vi "Rubbish.vi"() -> ()   [LabVIEW 2014]
uses:
  <vilib>/myRIO/Common/Instrument Driver Framework/myRIO v1.0/DIO/typedefs/DIO Channels Enum.ctl
  <vilib>/myRIO/Common/Instrument Driver Framework/myRIO v1.0/DIO/typedefs/DIO Channels List.ctl
  <vilib>/myRIO/Common/Instrument Driver Framework/Utilities/typedefs/Generic FPGA Reference.ctl
  <vilib>/myRIO/Common/Instrument Driver Framework/Utilities/typedefs/myRIO v1.0 Reference.ctl
  <vilib>/myRIO/Common/Instrument Driver Framework/Utilities/typedefs/Hardware Version Enum.ctl
  <vilib>/myRIO/Common/Instrument Driver Framework/Utilities/typedefs/myRIO Generic Hardware Reference.ctl
  <vilib>/myRIO/Instrument Drivers/Onboard IO/DIO/typedefs/DIO Reference.ctl
  <vilib>/myRIO/Instrument Drivers/Onboard IO/DIO/DIO.lvlib
  <vilib>/myRIO/Instrument Drivers/Onboard IO/DIO/vis/Read.vi
  <vilib>/userdefined/High Color/nirio_resource_hc.ctl
  <vilib>/myRIO/Common/Instrument Driver Framework/myRIO v1.0/DIO/vis/myRIO v1.1 Open DIO.vi
  <vilib>/myRIO/Instrument Drivers/Onboard IO/DIO/vis/myRIO DIO Open.xnode
  <vilib>/myRIO/Common/Instrument Driver Framework/Utilities/vis/Is FPGA Ref Available.vi
  <vilib>/myRIO/Express VI/Onboard IO/DI/DI Express VI.xnode
  <vilib>/functionblocks/Edge Detection/One Shot Falling With Input/One Shot Falling With Input.vi
  <vilib>/functionblocks/NI_FunctionBlock Libraries.lvlib
  <vilib>/functionblocks/FB Core/FB Core.xnode
  <vilib>/myRIO/Instrument Drivers/Onboard IO/DIO/vis/Write.vi
  <vilib>/myRIO/Express VI/Onboard IO/DO/DO Express VI.xnode
  <vilib>/myRIO/Instrument Drivers/Utilities/Utilities.lvlib
panel:
  in  "stop":bool
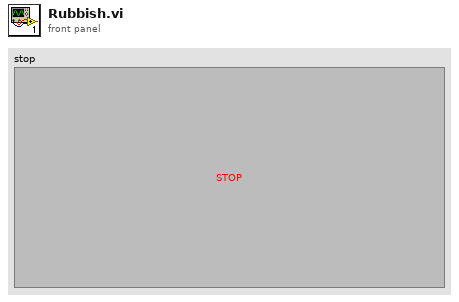
[diagram p1: front panel]
types:
  T1 = typedef "DIO.lvlib/DIO Reference.ctl" = cluster{"myRIO Reference":T2, "DIO Channels List":T6}
  T2 = typedef "myRIO Generic Hardware Reference.ctl" = cluster{"myRIO Model":T3, "myRIO Hardware Reference":T4}
  T3 = typedef "Hardware Version Enum.ctl" = enum16{"Unknown", "myRIO-1900", "myRIO-1950"}
  T4 = typedef "myRIO v1.0 Reference.ctl" = cluster{"Generic FPGA Reference":T5, "Allow multiple opens":bool}
  T5 = typedef "Generic FPGA Reference.ctl" = refnum<k20>
  T6 = typedef "DIO Channels List.ctl" = T7[]
  T7 = typedef "DIO Channels Enum.ctl" = enum16{"Not Connected", "C/DIO0", "C/DIO1", "C/DIO2", "C/DIO3", "C/DIO4", "C/DIO5", "C/DIO6", "C/DIO7", "A/DIO0", "A/DIO1", "A/DIO2", "A/DIO3", "A/DIO4", "A/DIO5", "A/DIO6", "A/DIO7", "A/DIO8", "A/DIO9", "A/DIO10", "A/DIO11", "A/DIO12", "A/DIO13", "A/DIO14", "A/DIO15", "B/DIO0", "B/DIO1", "B/DIO2", "B/DIO3", "B/DIO4", "B/DIO5", "B/DIO6", "B/DIO7", "B/DIO8", "B/DIO9", "B/DIO10", "B/DIO11", "B/DIO12", "B/DIO13", "B/DIO14", "B/DIO15", "LED0", "LED1", "LED2", "LED3", "Button0"}
  T8 = typedef "nirio_resource_hc.ctl" = tag
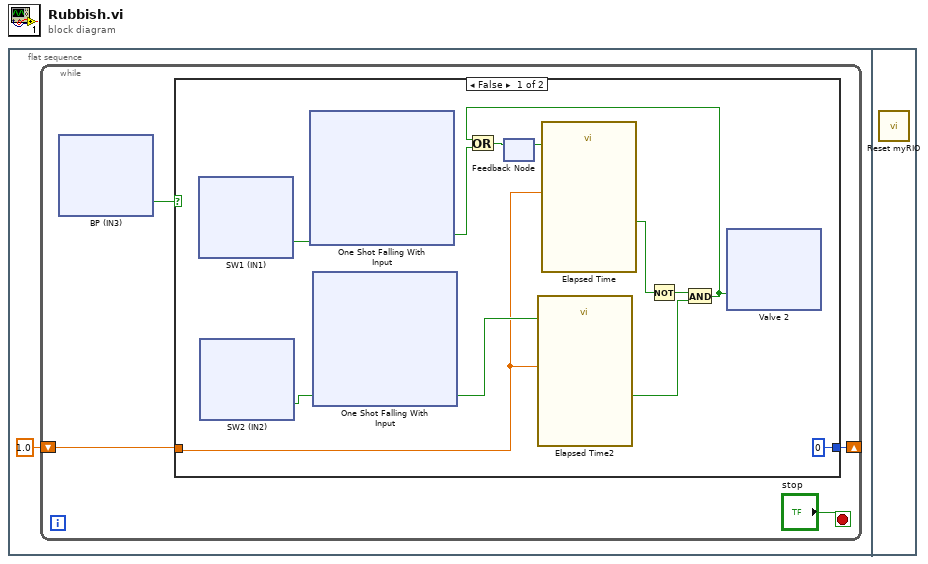
[diagram p0: block diagram]
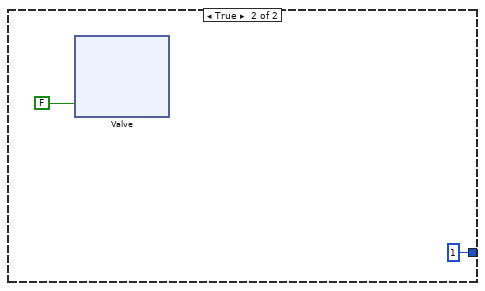
[diagram p2: hidden frame]
diagram:
  n1 = flat-sequence {
    frame #0 {
      n2 = while {
        shift-right: [w2] -> _
        shift-left: 1.0 -> [w3]
        stop <- "stop" stop-if-true
        n3 = xnode "BP (IN3)"() -> ("B/DIO1 (Pin 13)"=w4:bool)  [unwired: 1 in, 1 out]
        n4 = case shown="False" w4 {
          tunnel: w3 -> [w8 _]
          tunnel: [0 1] -> w2
          frame False {
            n5 = xnode "SW1 (IN1)"() -> ("B/DIO5 (Pin 21)"=w9:bool)  [unwired: 1 in, 1 out]
            n6 = xnode "SW2 (IN2)"() -> ("B/DIO2 (Pin 15)"=w17:bool)  [unwired: 1 in, 1 out]
            n7 = xnode "One Shot Falling With Input"("input"=w9) -> ("output"=w10:bool)  [unwired: 1 in, 1 out]
            n8 = xnode "One Shot Falling With Input"("input"=w17) -> ("output"=w14:bool)  [unwired: 1 in, 1 out]
            n9 = feedback #1() -> (w15:bool)  [unwired: 1 in]
            n10 = call "Elapsed Time2"("Reset"=w14, "Set Start Time (s)"=w8) -> ("Time has Elapsed"=w11:bool)  [unwired: 10 in, 7 out]
            n11 = call "Elapsed Time"("Reset"=w15, "Set Start Time (s)"=w8) -> ("Time has Elapsed"=w12:bool)  [unwired: 10 in, 7 out]
            n12 = Not(x=w12) -> (.not. x?=w13:bool)
            n13 = And(x=w13, y=w11) -> (x .and. y?=w6:bool)
            n14 = Or(x=w6, y=w10) -> (x .or. y?=w16:bool)
            n15 = feedback-in #1(w16) -> ()
            n16 = xnode "Valve 2"("A/DIO1 (Pin 13)"=w6) -> ()  [unwired: 1 in, 1 out]
          }
          frame True {
            n17 = xnode "Valve"("A/DIO1 (Pin 13)"=FALSE) -> ()  [unwired: 1 in, 1 out]
          }
        }
      }
    }
    frame #1 {
      n18 = call <vilib>:"Reset myRIO.vi"() -> ()  [unwired: 11 in, 1 out]
    }
  }
